vi "MixAndDownsample_5782.vi"(4 "sin1":fxp<+/-,16,0>, 6 "sin0":fxp<+/-,16,0>, 8 "cos1":fxp<+/-,16,0>, 9 "cos0":fxp<+/-,16,0>, 10 "signal 1":i16, 11 "signal 0":i16) -> (0 "data valid":bool, 1 "Q out":fxp<+/-,16,14>, 2 "I out":fxp<+/-,16,14>)   [LabVIEW 2013]
uses:
  <vilib>/rvi/FXPMathLib/FxpSub/XNode/nifxpmath_Sub.xnode
  <vilib>/rvi/FXPMathLib/sim/FxpSim.dll
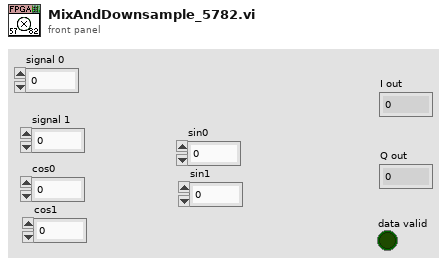
[diagram p1: front panel]
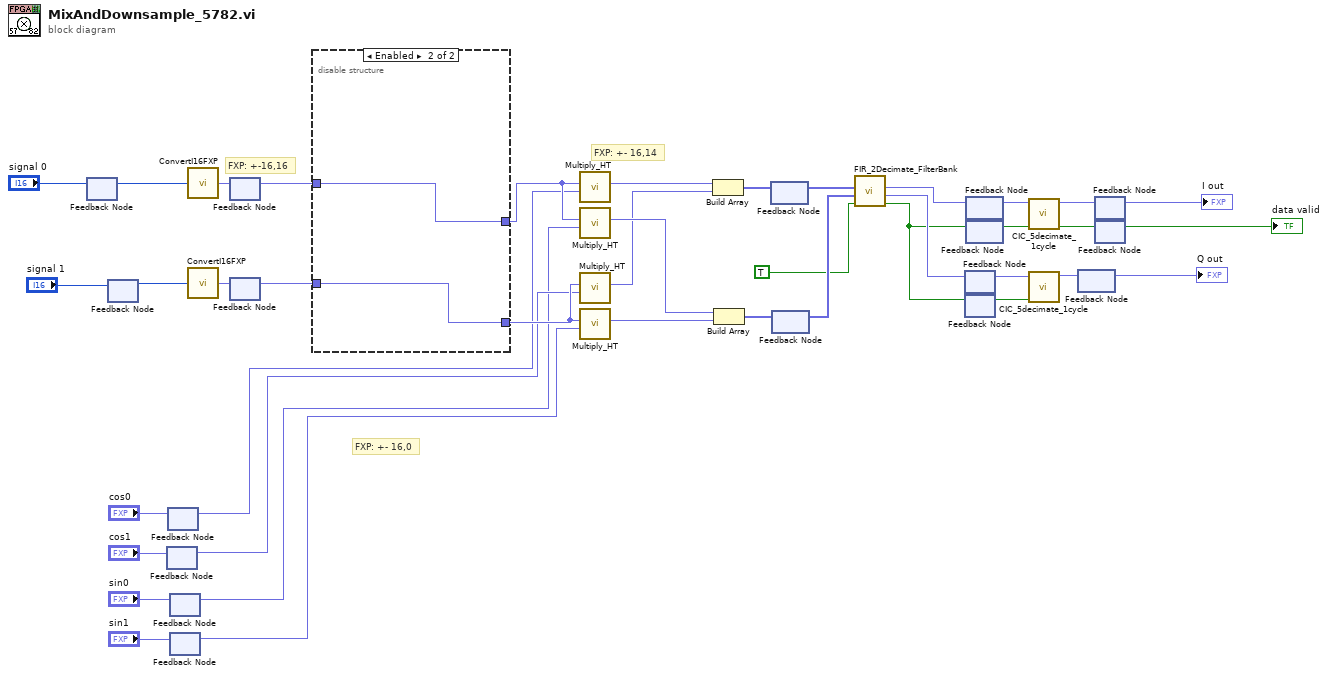
[diagram p0: block diagram]
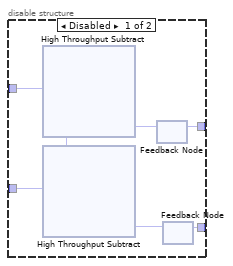
[diagram p2: hidden frame]
diagram:
  # "FXP: +- 16,14"
  # "FXP: +- 16,0"
  # "FXP: +-16,16"
  n1 = feedback #1() -> (w11:i16)  [unwired: 1 in]
  n2 = feedback-in #1("signal 0") -> ()
  n3 = feedback #2() -> (w10:i16)  [unwired: 1 in]
  n4 = feedback-in #2("signal 1") -> ()
  n5 = feedback #3() -> (w3:fxp<+/-,16,0>)  [unwired: 1 in]
  n6 = feedback-in #3("cos1") -> ()
  n7 = feedback #4() -> (w4:fxp<+/-,16,0>)  [unwired: 1 in]
  n8 = feedback-in #4("cos0") -> ()
  n9 = feedback #5() -> (w2:fxp<+/-,16,0>)  [unwired: 1 in]
  n10 = feedback-in #5("sin0") -> ()
  n11 = feedback #6() -> (w1:fxp<+/-,16,0>)  [unwired: 1 in]
  n12 = feedback-in #6("sin1") -> ()
  n13 = call "ConvertI16FXP.vi"("I16"=w11) -> ("y"=w30:fxp<+/-,16,16>)
  n14 = call "ConvertI16FXP.vi"("I16"=w10) -> ("y"=w29:fxp<+/-,16,16>)
  n15 = feedback #7() -> (w16:fxp<+/-,16,16>)  [unwired: 1 in]
  n16 = feedback-in #7(w30) -> ()
  n17 = feedback #8() -> (w15:fxp<+/-,16,16>)  [unwired: 1 in]
  n18 = feedback-in #8(w29) -> ()
  n19 = disable-structure shown="Enabled" {
    disable-tunnel: w16 -> [w47 w49]
    disable-tunnel: w15 -> [w46 w48]
    disable-tunnel: [w43 w49] -> w14
    disable-tunnel: [w41 w48] -> w13
    frame Disabled {
      n20 = xnode "High Throughput Subtract"("x"=w47) -> ("y"=w45:fxp<+/-,16,16>, "x-y"=w44:fxp<+/-,16,16>)
      n21 = xnode "High Throughput Subtract"("x"=w46, "y"=w45) -> ("x-y"=w42:fxp<+/-,16,16>)
      n22 = feedback #9() -> (w43:fxp<+/-,16,16>)  [unwired: 1 in]
      n23 = feedback-in #9(w44) -> ()
      n24 = feedback #10() -> (w41:fxp<+/-,16,16>)  [unwired: 1 in]
      n25 = feedback-in #10(w42) -> ()
    }
    frame Enabled {
    }
  }
  n26 = call "Multiply_HT.vi"("DDS sample"=w4, "Signal sample"=w14) -> ("Output"=w28:fxp<+/-,16,14>)  [unwired: 8 in, 1 out]
  n27 = call "Multiply_HT.vi"("DDS sample"=w2, "Signal sample"=w14) -> ("Output"=w27:fxp<+/-,16,14>)  [unwired: 8 in, 1 out]
  n28 = call "Multiply_HT.vi"("DDS sample"=w3, "Signal sample"=w13) -> ("Output"=w26:fxp<+/-,16,14>)  [unwired: 8 in, 1 out]
  n29 = call "Multiply_HT.vi"("DDS sample"=w1, "Signal sample"=w13) -> ("Output"=w25:fxp<+/-,16,14>)  [unwired: 8 in, 1 out]
  n30 = Build Array(w28, w26) -> (w24:fxp<+/-,16,14>[])
  n31 = Build Array(w27, w25) -> (w23:fxp<+/-,16,14>[])
  n32 = feedback #11() -> (w22:fxp<+/-,16,14>[])  [unwired: 1 in]
  n33 = feedback-in #11(w24) -> ()
  n34 = feedback #12() -> (w21:fxp<+/-,16,14>[])  [unwired: 1 in]
  n35 = feedback-in #12(w23) -> ()
  n36 = call "FIR_2Decimate_FilterBank.vi"("data valid in"=TRUE ("valid in"), "Q in"=w21, "I in"=w22) -> ("data valid out"=w17:bool, "Q out"=w18:fxp<+/-,16,14>, "I out"=w19:fxp<+/-,16,14>)  [unwired: 6 in]
  n37 = feedback #13() -> (w36:fxp<+/-,16,14>)  [unwired: 1 in]
  n38 = feedback-in #13(w18) -> ()
  n39 = feedback #14() -> (w35:bool)  [unwired: 1 in]
  n40 = feedback-in #14(w17) -> ()
  n41 = feedback-in #15(w19) -> ()
  n42 = feedback #15() -> (w40:fxp<+/-,16,14>)  [unwired: 1 in]
  n43 = feedback #16() -> (w39:bool)  [unwired: 1 in]
  n44 = feedback-in #16(w17) -> ()
  n45 = call "CIC_5decimate_1cycle.vi"("valid in"=w39, "Data in"=w40) -> ("valid out"=w32:bool, "Data out"=w34:fxp<+/-,16,14>)  [unwired: 8 in]
  n46 = call "CIC_5decimate_1cycle.vi"("valid in"=w35, "Data in"=w36) -> ("Data out"=w38:fxp<+/-,16,14>)  [unwired: 8 in, 1 out]
  n47 = feedback #17() -> (→"Q out":fxp<+/-,16,14>)  [unwired: 1 in]
  n48 = feedback-in #17(w38) -> ()
  n49 = feedback #18() -> (→"I out":fxp<+/-,16,14>)  [unwired: 1 in]
  n50 = feedback-in #18(w34) -> ()
  n51 = feedback #19() -> (→"data valid":bool)  [unwired: 1 in]
  n52 = feedback-in #19(w32) -> ()
